vi "Create and Save Project.vi"(0 "Project Path":path=path "D:/Reference Architecture/Test.lvproj", 11 "error in (no error)":errorcluster) -> (15 "error out":errorcluster)   [LabVIEW 2021, in "Migrator.lvlib"]
uses:
  Migrator.lvlib
  Path Functions/Path Functions.lvlib
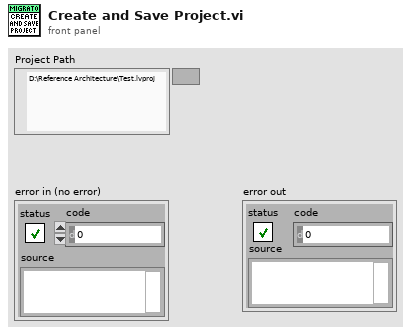
[diagram p1: front panel]
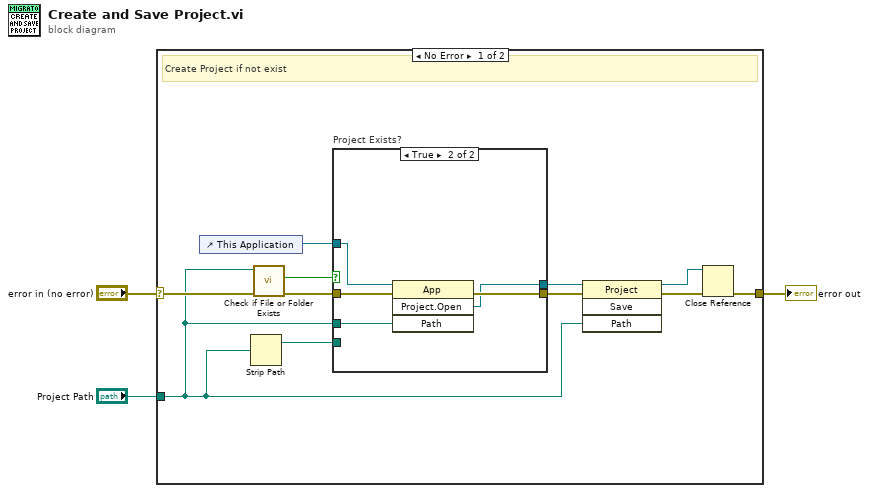
[diagram p0: block diagram]
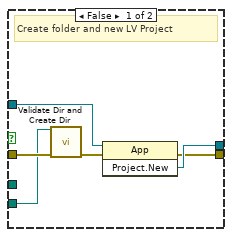
[diagram p2: hidden frame]
diagram:
  n1 = case shown="No Error" "error in (no error)" {
    selector: "error in (no error)" -> [w13 w26]
    tunnel: "Project Path" -> [w10 _]
    tunnel: [w5 w26] -> w1
    frame No Error {
      # "Create Project if not exist"
      n2 = control-ref of="This Application"() -> (w9:refnum<vi>)
      n3 = Strip Path(path=w10) -> (stripped path=w14:path)  [unwired: 1 out]
      n4 = call <vilib>:"Check if File or Folder Exists.vi"("error in (no error)"=w13, "path"=w10) -> ("error out"=w12:errorcluster, "file or folder exists?"=w11:bool)  [unwired: 7 in, 1 out]
      n5 = case "Project Exists?" shown="True" w11 {
        tunnel: [w20 w22] -> w8
        tunnel: [w19 w23] -> w7
        tunnel: w14 -> [w16 _]
        tunnel: w12 -> [w17 w25]
        tunnel: w10 -> [_ w24]
        tunnel: w9 -> [w18 w21]
        frame False {
          # "Create folder and new LV Project"
          n6 = call "Validate Dir and Create Dir.vi"("Directory"=w16, "error in (no error)"=w17) -> ("error out"=w15:errorcluster)  [unwired: 12 in, 1 out]
          n7 = invoke class="App" method="Project.New"(reference=w18, error in=w15) -> (error out=w19:errorcluster, "Project:New"=w20:refnum<vi>)  [unwired: 1 in, 1 out]
        }
        frame True {
          n8 = invoke class="App" method="Project.Open"(reference=w21, error in=w25, "Path"=w24) -> (error out=w23:errorcluster, "Project:Open"=w22:refnum<vi>)  [unwired: 1 in, 2 out]
        }
      }
      n9 = invoke class="Project" method="Save"(reference=w8, error in=w7, "Path"=w10) -> (reference out=w4:refnum<vi>, error out=w6:errorcluster)  [unwired: 1 in, 2 out]
      n10 = Close Reference(reference=w4, error in (no error)=w6) -> (error out=w5:errorcluster)
    }
    frame Error {
    }
  }
  "error out" <- w1
